vi "Read Test.vi"(11 "Executioner in":refnum<class "Executioner.lvclass">) -> (3 "Executioner out":refnum<class "Executioner.lvclass">, 4 "Test":string)   [LabVIEW 2019, in "Test Executive.lvlib" / "Executioner.lvclass"]
uses:
  <vilib>/gpm_packages/@cs/test-executive/Source/Test Executive/Executioner/Executioner.lvclass
  <vilib>/gpm_packages/@cs/test-executive/Source/Test Executive/Executioner/Executioner.lvclass/Executioner.ctl
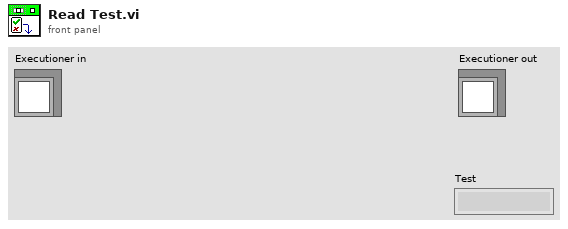
[diagram p1: front panel]
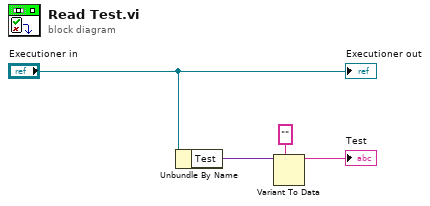
[diagram p0: block diagram]
diagram:
  n1 = Unbundle By Name("Executioner in") -> ("Test"=w2:variant)
  n2 = Variant To Data(type="", Variant=w2) -> (data=→"Test":string)  [unwired: 1 in, 1 out]
  "Executioner out" <- "Executioner in"
